vi "OAT CIC Interpolator Decimator Design.vi"(9 "lag":i32=1, 10 "stages":i32=2, 11 "interpolation/decimation factor":i32=2) -> (0 "error out":errorcluster, 1 "filter":T1={"coefficients"=[], "factor"=1} {"coefficients" format="%.2f"})   [LabVIEW 2017, in "SoundVib_Resampling.lvlib"]
doc: "Design a single stage interpolation/decimation filter based on CIC filter"
uses:
  <vilib>/addons/Sound and Vibration/Order Analysis/Resample Order Tracking/SoundVib_Resampling.lvlib
  <vilib>/addons/_NISVFA/_Shared subVIs/Controls/OAT Decimation Filter.ctl
  <vilib>/Analysis/2dsp.llb/1D Convolution (DBL).vi
  <vilib>/Analysis/NI_AALPro.lvlib
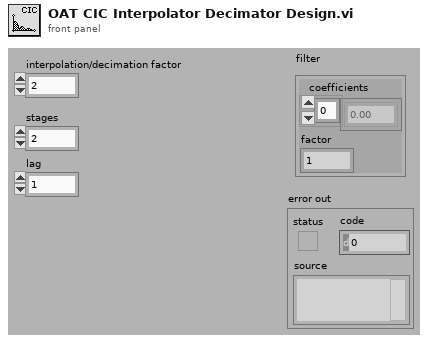
[diagram p1: front panel]
types:
  T1 = typedef "OAT Decimation Filter.ctl" = cluster{"coefficients":dbl[], "factor":i32}
  T2 = cluster{"stages":i32, "interpolation/decimation factor":i32, "lag":i32}
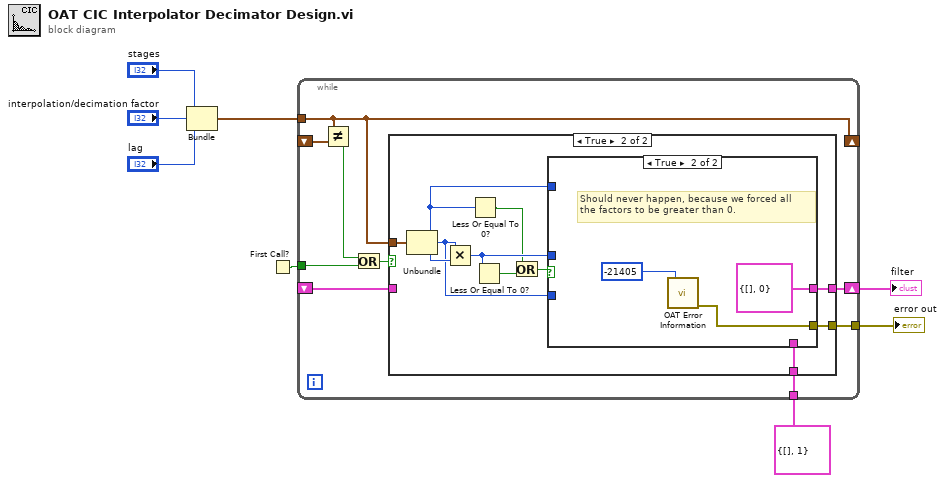
[diagram p0: block diagram]
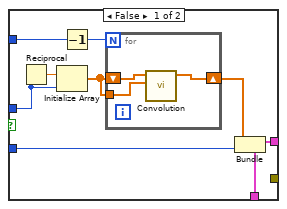
[diagram p3: hidden frame]
diagram:
  n1 = Bundle("stages"="stages", "interpolation/decimation factor"="interpolation/decimation factor", "lag"="lag") -> (w1:T2)  [unwired: 1 in]
  n2 = First Call?() -> (First Call?: T/F=w8:bool)
  n3 = while {
    tunnel: w8 -> [w14]
    shift-left: _ -> [w12]
    shift-right: [w11] -> _
    shift-left: _ -> [w16]
    shift-right: [w17] -> w7
    tunnel: w1 -> [w11]
    tunnel: T1 {"coefficients"=[], "factor"=1} ("filter") -> [w10]
    tunnel: [w9] -> w2
    stop <- FALSE continue-if-true
    n4 = Not Equal?(x=w11, y=w12) -> (x != y?=w13:bool)
    n5 = Or(x=w13, y=w14) -> (x .or. y?=w15:bool)
    n6 = case shown="True" w15 {
      tunnel: [w19 w29] -> w17
      tunnel: w11 -> [_ w30]
      tunnel: w16 -> [w19 _]
      tunnel: w10 -> [_ w26]
      tunnel: [_ w24] -> w9
      frame False {
      }
      frame True {
        n7 = Unbundle(w30) -> ("stages"=w23:i32, "interpolation/decimation factor"=w27:i32, "lag"=w28:i32)
        n8 = Multiply(x=w27, y=w28) -> (x*y=w25:i32)
        n9 = Less Or Equal To 0?(x=w23) -> (x <= 0?=w21:bool)
        n10 = Less Or Equal To 0?(x=w25) -> (x <= 0?=w22:bool)
        n11 = Or(x=w21, y=w22) -> (x .or. y?=w20:bool)
        n12 = case shown="True" w20 {
          tunnel: [w39 T1 {"coefficients"=[], "factor"=0} ("filter")] -> w29
          tunnel: w23 -> [w34 _]
          tunnel: w27 -> [w33 _]
          tunnel: w26 -> [w32 _]
          tunnel: w25 -> [w31 _]
          tunnel: [_ w43] -> w24
          frame False {
            n13 = Reciprocal(x=w31) -> (1/x=w37:dbl)
            n14 = Initialize Array(w37, w31) -> (w36:dbl[])
            n15 = Decrement(x=w34) -> (x-1=w38:i32)
            n16 = for {
              N: w38 -> [_]
              shift-right: [w41] -> w35
              shift-left: w36 -> [w42]
              tunnel: w36 -> [w40]
              n17 = call-poly <vilib>:"Convolution.vi"("Y"=w40, "X"=w42) -> ("X * Y"=w41:dbl[])  [unwired: 8 in, 1 out]
            }
            n18 = Bundle(cluster=w32, "coefficients"=w35, "factor"=w33) -> (w39:T1)
          }
          frame True {
            # "Should never happen, because we forced all \nthe factors to be greater than 0."
            n19 = call <vilib>:"OAT Error Information.vi"("error code"=-21405) -> ("error out"=w43:errorcluster)  [unwired: 6 in]
          }
        }
      }
    }
  }
  "filter" <- w7
  "error out" <- w2
